vi "PicoScope3000aExampleStreamingAdvancedTrig.vi"() -> ()   [LabVIEW 2010]
doc: "This example demonstrates how to use the PicoScope Labview library to stream data from a PicoScope 5000 Series Device"
uses:
  <vilib>/Waveform/DWDTOps.llb/DWDT Analog to Digital.vi
  ps3000aWrap.dll
  PicoScope3000aLib/PicoScope3000aAnalogChannelSettings.ctl
  PicoScope3000aLib/PicoScope3000aDigitalChannelSettings.ctl
panel:
  in  "Write ChA to file":bool
  in  "Pulse Width Qualifier Conditions":T1 {"Condition Logic" items=["AND", "OR", "XOR"]}
  in  "Digital Port  0":T2 {"Direction Channel 7" items=["Don't Care", "Low", "High", "Rising", "Falling"]; "Direction Channel 6" items=["Don't Care", "Low", "High", "Rising", "Falling"]; "Direction Channel 5" items=["Don't Care", "Low", "High", "Rising", "Falling"]; "Direction Channel 4" items=["Don't Care", "Low", "High", "Rising", "Falling"]; "Direction Channel 3" items=["Don't Care", "Low", "High", "Rising", "Falling"]; "Direction Channel 2" items=["Don't Care", "Low", "High", "Rising", "Falling"]; "Direction Channel 1" items=["Don't Care", "Low", "High", "Rising", "Falling"]; "Direction Channel 0" items=["Don't Care", "Low", "High", "Rising", "Falling"]}
  in  "Pulse Width Qualifier Settings":T3={"Direction"=2, "Lower Limit"=0, "Upper Limit"=0, "Pulse Width Type"=0} {"Pulse Width Type" items=["None", "Less Than", "Greater Than", "In Range", "Out of Range"]; "Direction" items=["Rising"=2, "Falling"=3]}
  in  "Auto Trigger (ms)":i32=1000
  in  "Trigger Conditions":T4 {"Condition Logic" items=["AND", "OR", "XOR"]}
  in  "Channel B Trigger Properties":T5={"thresholdUpper"=0, "thresholdUpperHysteresis"=1024, "thresholdLower"=0, "thresholdLowerHysteresis"=1024, "Threshold Mode"=0, "Direction"=2, "Available"=FALSE} {"Direction" items=["Above / Inside", "Below / Outside", "Rising / Enter", "Falling / Exit", "Rising or Falling / Enter or Exit", "Above Lower", "Below Lower", "Rising Lower", "Falling Lower", "Positive Runt", "Negative Runt"]; "Threshold Mode" items=["Level", "Window"]}
  in  "Channel A Trigger Properties":T5={"thresholdUpper"=0, "thresholdUpperHysteresis"=1024, "thresholdLower"=0, "thresholdLowerHysteresis"=1024, "Threshold Mode"=0, "Direction"=2, "Available"=FALSE} {"Direction" items=["Above / Inside", "Below / Outside", "Rising / Enter", "Falling / Exit", "Rising or Falling / Enter or Exit", "Above Lower", "Below Lower", "Rising Lower", "Falling Lower", "Positive Runt", "Negative Runt"]; "Threshold Mode" items=["Level", "Window"]}
  in  "Port 0 Settings":T6={"Enabled"=FALSE, "Logic Level"=9830} {"Logic Level" items=["1.5V TTL"=9830, "2.5V CMOS"=16383]}
  in  "Channel A Settings":T7={"Enabled"=TRUE, "Coupling"=1, "Range"=6, "Analogue Offset"=0.0, "Bandwidth Limit"=0} {"Bandwidth Limit" items=["Full", "20MHz"]; "Range" items=["10 mV", "20 mV", "50 mV", "100 mV", "200 mV", "500 mV", "1 V", "2 V", "5 V", "10 V", "20 V", "50 V ", "100 V"]; "Coupling" items=["AC", "DC"]}
  out "Analog Channels":T8(graph)
  out "Raw Sample Interval (sec)":dbl=1.0000000130088963e-06 format="%#.5p"
  out "Max ADC value":i16
  out "Chunk time":u32
  out "Elapsed time":dbl
  in  "Data file":path=path "PicoScope3000aExampleStreaming ChA Data"
  out "size(s)":i32
  out "Queue depth":i32(graph)
  out "queue depth":i32
  in  "Buffer and Transfer Settings":T9={"startIndex"=0, "Samples"=1000000, "Down Sample Ratio"=1, "Down-Sample Mode"=0} {"Down-Sample Mode" items=["None"=0, "Aggregate"=1, "Decimate"=2, "Average"=4]; "Down Sample Ratio" step=1; "Samples" format="%_6p"}
  out "USB Powered":bool=TRUE
  out "USB 3.0 device on non-USB 3.0 Port":bool=TRUE
  out "TriggeredAt (In Buffer)":u32 format="%#.6p"
  out "TriggeredAt (Total samples)":u32 format="%#.6p"
  in  "Acquisition Settings":T10={"Auto Stop"=TRUE, "Desired Sample Interval"=1, "Pre-trigger Samples"=500000, "Post-trigger Samples"=500000, "Down-Sample Ratio"=1, "Down-Sample Mode"=0, "Time Units"=3} {"Time Units" items=["Nanoseconds (ns)"=2, "Microseconds (us)"=3, "Milliseconds (ms)"=4, "Seconds (s)"=5]; "Down-Sample Mode" items=["None"=0, "Aggregate"=1, "Decimate"=2, "Average"=4]; "Post-trigger Samples" format="%#.6p"; "Pre-trigger Samples" format="%#_6p"}
  out "Port 0":digitalwaveform(graph)={"t0"=timestamp(0 s since 1904-01-01), "dt"=1.0000000130088963e-06, "Y"={"transitions"=[], "data"=[]}}
  out "Triggered":bool
  out "DownSample Interval (sec)":dbl=1.0000000130088963e-06 format="%#.5p"
  out "Total Samples":u32 format="%#.6p"
  out "Auto Stopped":bool
  in  "Serial Number":string
  in  "Open Using Serial Number":bool
  out "Number of Samples per Capture":u32 format="%#.6p"
  in  "Apply  Settings":bool
  in  "stop":bool
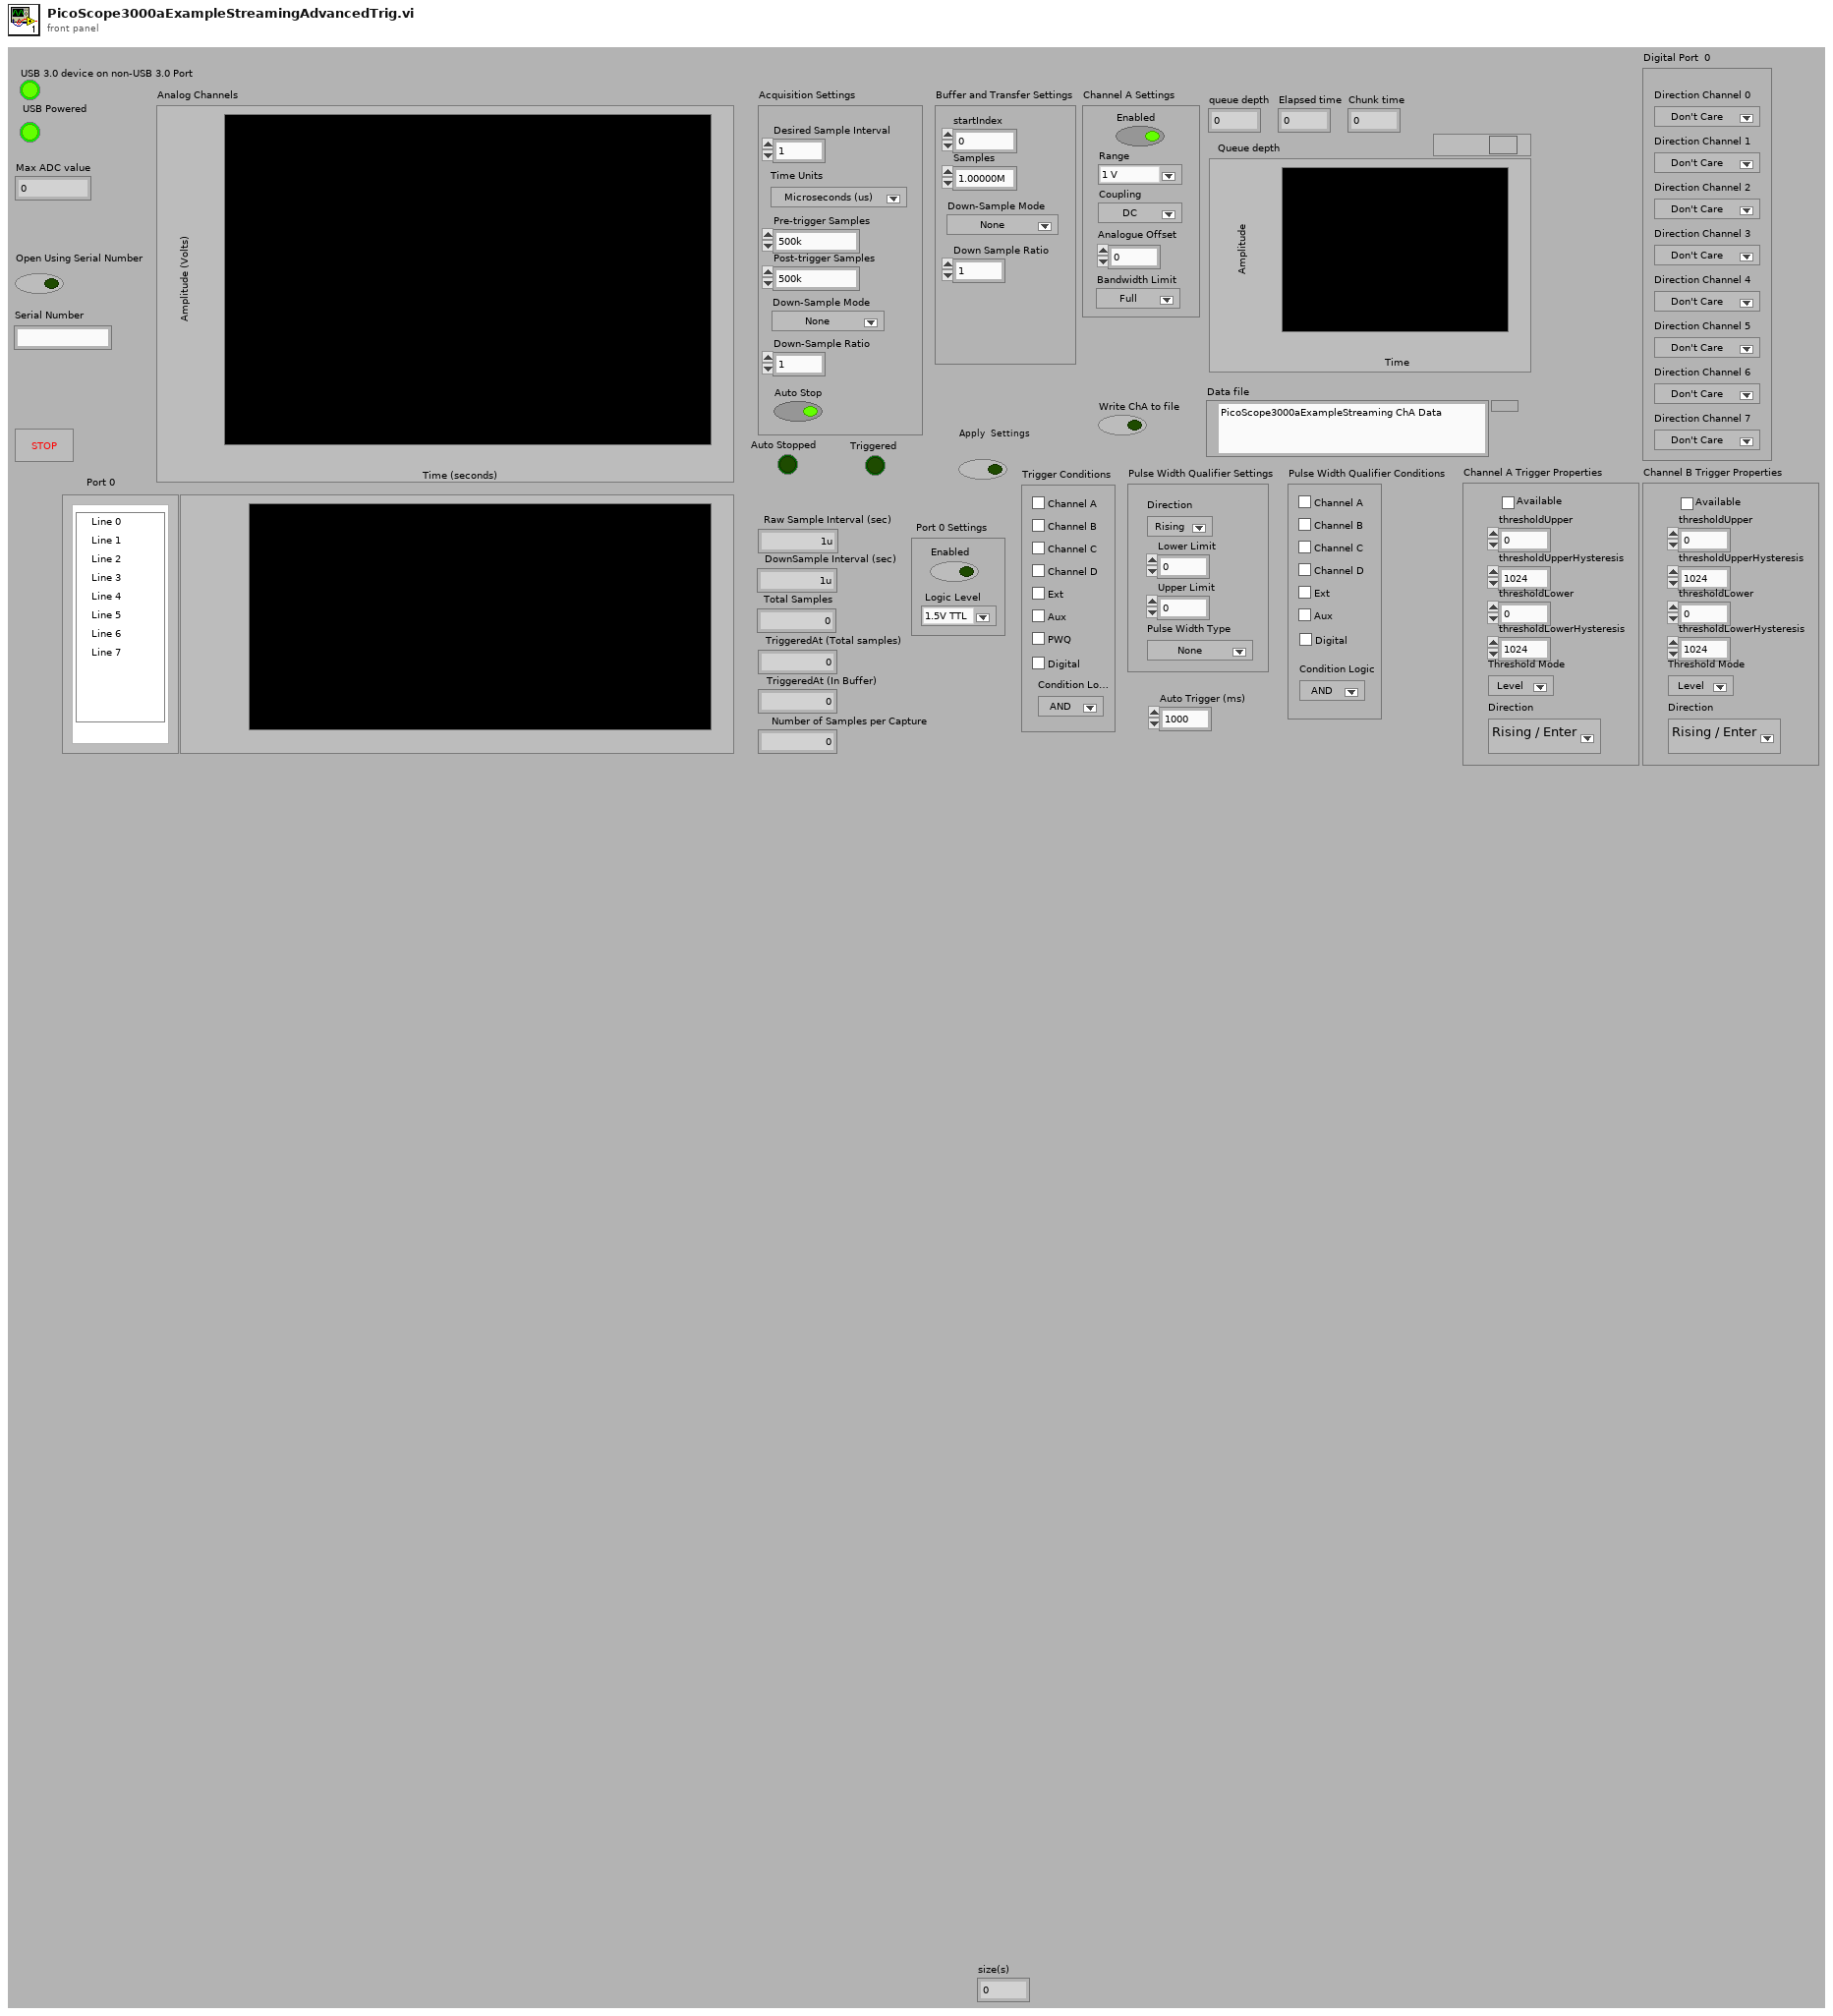
[diagram p1: front panel]
types:
  T1 = cluster{"Channel A":bool, "Channel B":bool, "Channel C":bool, "Channel D":bool, "Aux":bool, "Condition Logic":u16, "Ext":bool, "Digital":bool}
  T2 = cluster{"Direction Channel 0":u16, "Direction Channel 1":u16, "Direction Channel 2":u16, "Direction Channel 3":u16, "Direction Channel 4":u16, "Direction Channel 5":u16, "Direction Channel 6":u16, "Direction Channel 7":u16}
  T3 = cluster{"Direction":u32, "Lower Limit":u32, "Upper Limit":u32, "Pulse Width Type":u32}
  T4 = cluster{"Channel A":bool, "Channel B":bool, "Channel C":bool, "Channel D":bool, "Aux":bool, "PWQ":bool, "Condition Logic":u16, "Ext":bool, "Digital":bool}
  T5 = cluster{"thresholdUpper":i16, "thresholdUpperHysteresis":u16, "thresholdLower":i16, "thresholdLowerHysteresis":u16, "Threshold Mode":i32, "Direction":i32, "Available":bool}
  T6 = typedef "PicoScope3000aDigitalChannelSettings.ctl" = cluster{"Enabled":bool, "Logic Level":i16}
  T7 = typedef "PicoScope3000aAnalogChannelSettings.ctl" = cluster{"Enabled":bool, "Coupling":u32, "Range":u32, "Analogue Offset":sgl, "Bandwidth Limit":u32}
  T8 = cluster{i32, "DownSample Interval (sec)":dbl, "Data":dbl[]}
  T9 = cluster{"startIndex":u64, "Samples":u64, "Down Sample Ratio":u64, "Down-Sample Mode":u32}
  T10 = cluster{"Auto Stop":bool, "Desired Sample Interval":u32, "Pre-trigger Samples":u32, "Post-trigger Samples":u32, "Down-Sample Ratio":u32, "Down-Sample Mode":i32, "Time Units":u32}
  T11 = enum16{"open", "open or create", "create or replace", "create", "open (read-only)"}
  T12 = cluster{"Driver Version":string, "USB Version":string, "Hardware":string, "Variant":string, "Batch and Serial":string, "Cal Date":string, "Kernel Version":string, "Digital HW Version":string, "Analogue HW Version":string, "MSO":bool, "Number of channels":i16}
  T13 = cluster{"Channel A Buffer":i16[], "Channel B Buffer":i16[], "Channel C Buffer":i16[], "Channel D Buffer":i16[], "Channel E Buffer":i16[], "Channel F Buffer":i16[], "Channel G Buffer":i16[], "Channel H Buffer":i16[], "Port 0":i16[], "Port 1":i16[]}
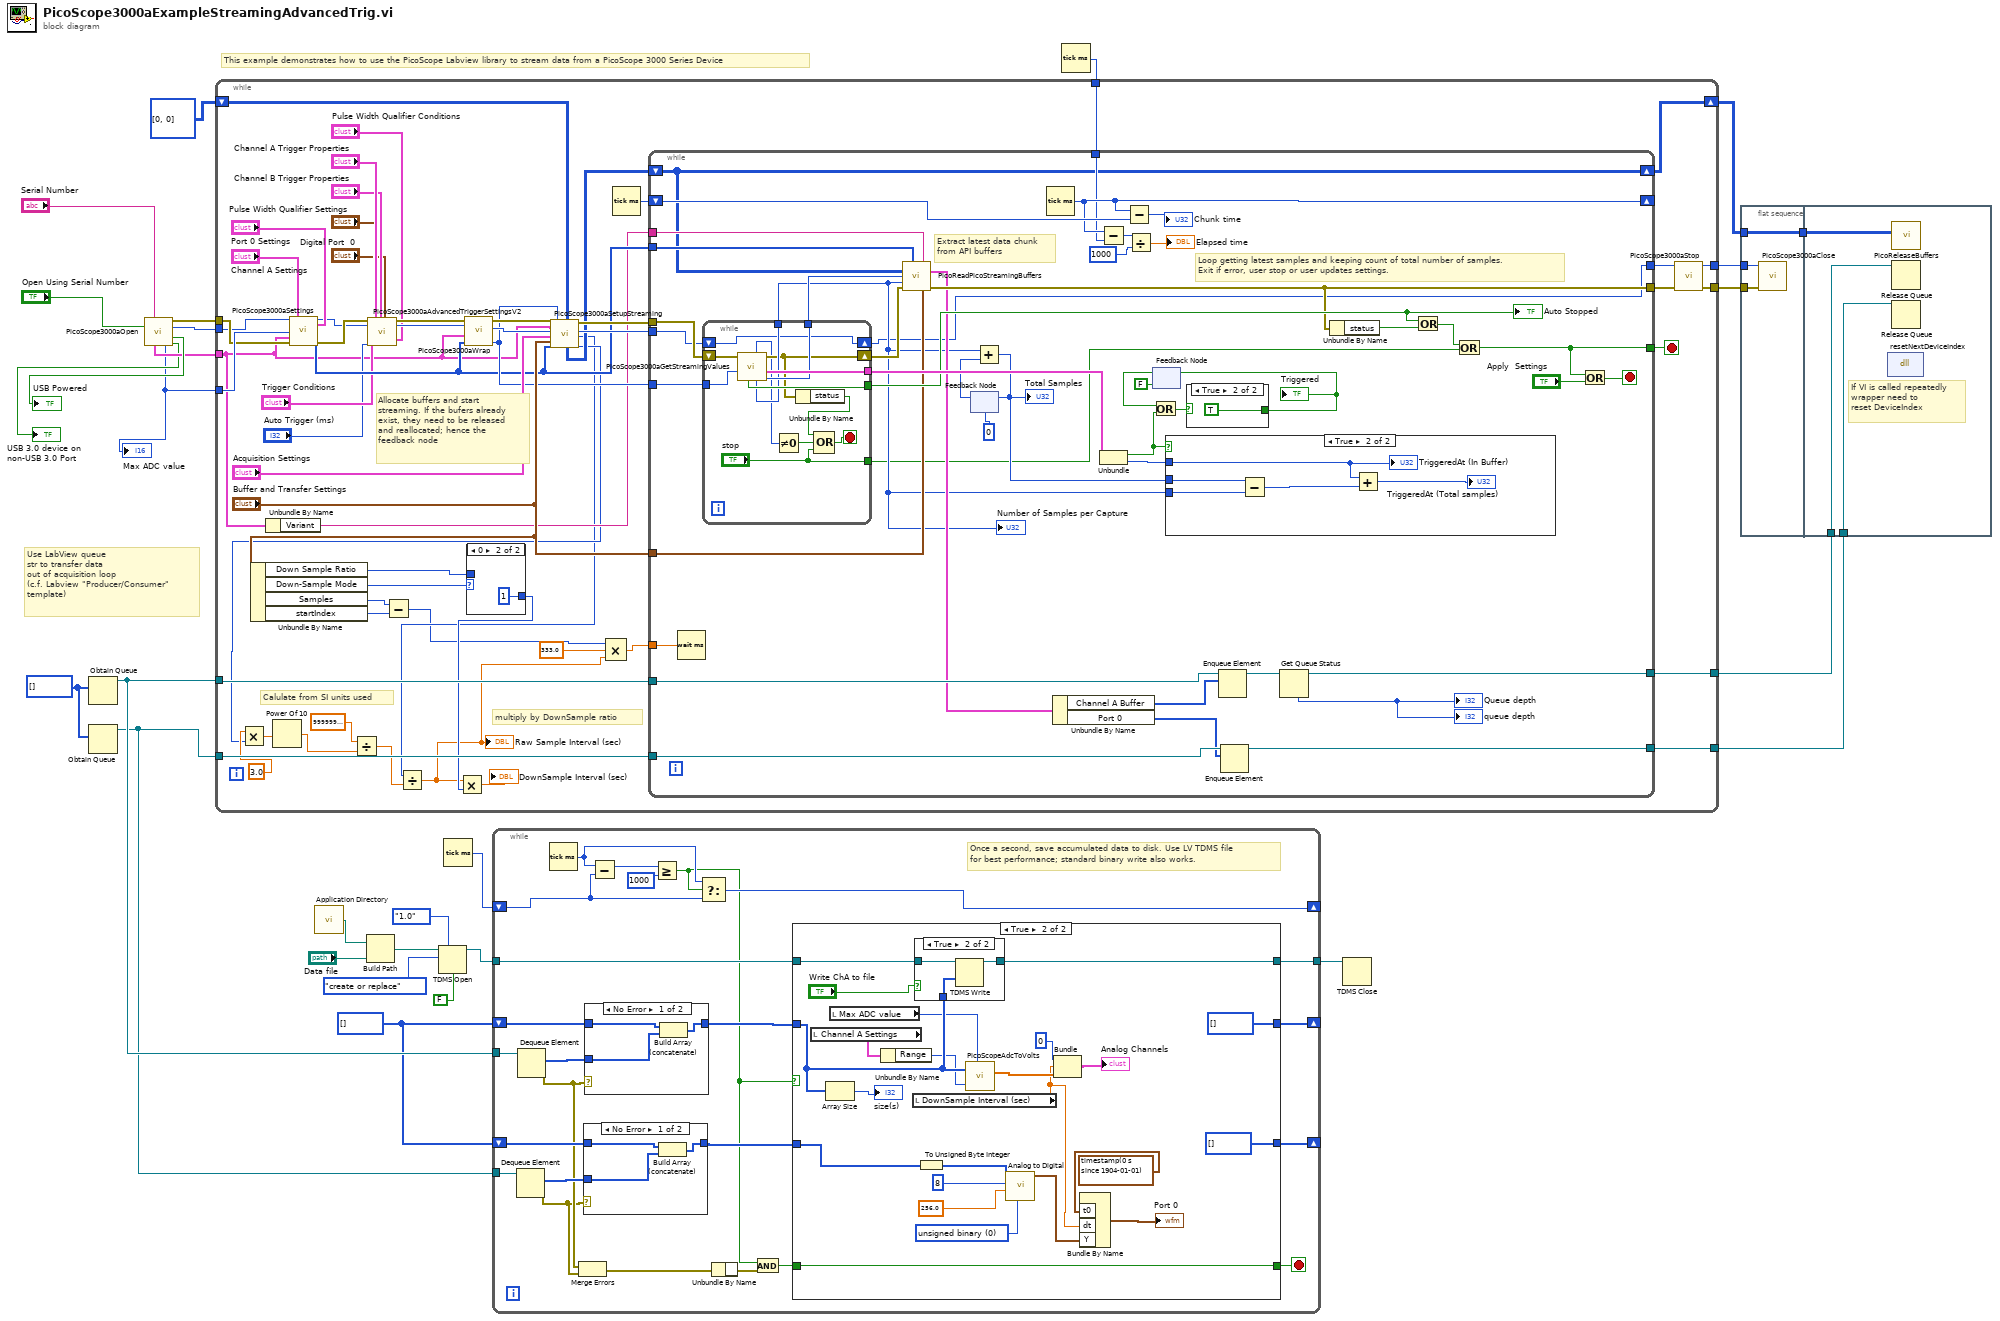
[diagram p0: block diagram]
diagram:
  w12 = i16[] [] ("History Data")
  w15 = i16[] [] ("History Data")
  # "Use LabView queue\nstr to transfer data\nout of acquisition loop\n(c.f. Labview \"Producer/Consumer\"\ntemplate)"
  # "This example demonstrates how to use the PicoScope Labview library to stream data from a PicoScope 3000 Series Device"
  n1 = Obtain Queue(element data type=w15) -> (queue out=w25:refnum<queue>)  [unwired: 4 in, 2 out]
  n2 = Obtain Queue(element data type=w15) -> (queue out=w13:refnum<queue>)  [unwired: 4 in, 2 out]
  n3 = call "PicoScope3000aOpen.vi"("Serial Number"="Serial Number", "Use Serial number"="Open Using Serial Number") -> ("error out"=w29:errorcluster, "handle"=w28:i16, "USB Powered"=→"USB Powered":bool, "Device Info"=w8:T12, "Max ADC value"=w6:i16, "USB 3.0 device on non-USB 3.0 Port"=→"USB 3.0 device on non-USB 3.0 Port":bool)  [unwired: 7 in, 1 out]
  "Max ADC value" <- w6
  n4 = call <vilib>:"Application Directory.vi"() -> ("Application Directory"=w9:path)
  n5 = Build Path(base path=w9, name or relative path="Data file") -> (appended path=w10:path)
  n6 = TDMS Open(6:FALSE ("disable buffering? (T)"), 7:enum16{"1.0", "2.0"}."1.0" ("file format version (2.0)"), 10:T11."create or replace" ("operation (0:open)"), 11:w10) -> (3:w19:refnum<k34>)  [unwired: 2 in, 1 out]
  n7 = Tick Count (ms)() -> (millisecond timer value=w21:u32)
  n8 = while {
    tunnel: w25 -> [w52]
    shift-right: [w44] -> _
    shift-left: w12 -> [w51]
    shift-right: [w46] -> _
    shift-left: w21 -> [w47]
    tunnel: w19 -> [w43]
    tunnel: [w42] -> w18
    tunnel: w13 -> [w40]
    shift-right: [w37] -> _
    shift-left: w12 -> [w39]
    stop <- w34 stop-if-true
    # "Once a second, save accumulated data to disk. Use LV TDMS file\nfor best performance; standard binary write also works."
    n9 = Dequeue Element(queue=w40) -> (element=w41:i16[], error out=w35:errorcluster)  [unwired: 2 in, 2 out]
    n10 = Dequeue Element(queue=w52) -> (element=w53:i16[], error out=w36:errorcluster)  [unwired: 2 in, 2 out]
    n11 = Tick Count (ms)() -> (millisecond timer value=w48:u32)
    n12 = Merge Errors(w36, w35) -> (w33:errorcluster)
    n13 = case shown="No Error" w35 {
      tunnel: w39 -> [w56 w57]
      tunnel: [w55 w57] -> w38
      tunnel: w41 -> [w54 _]
      frame No Error {
        n14 = Build Array (concatenate)(w56, w54) -> (w55:i16[])
      }
      frame Error {
      }
    }
    n15 = case shown="No Error" w36 {
      tunnel: w51 -> [w91 w92]
      tunnel: [w90 w92] -> w45
      tunnel: w53 -> [w89 _]
      frame No Error {
        n16 = Build Array (concatenate)(w91, w89) -> (w90:i16[])
      }
      frame Error {
      }
    }
    n17 = Subtract(x=w48, y=w47) -> (x-y=w50:u32)
    n18 = Greater Or Equal?(x=w50, y=u32 1000) -> (x >= y?=w31:bool)
    n19 = Select(t=w48, s=w31, f=w47) -> (s? t:f=w46:u32)
    n20 = And(x=w31) -> (y=w30:errorcluster, x .and. y?=w32:bool)
    n21 = Unbundle By Name(w33, w30) -> ()
    n22 = case shown="True" w31 {
      tunnel: w45 -> [w61 w80]
      tunnel: [w61 i16[] [] ("History Data")] -> w44
      tunnel: w43 -> [w60 w82]
      tunnel: [w60 w81] -> w42
      tunnel: w38 -> [w59 w67]
      tunnel: [w59 i16[] [] ("History Data")] -> w37
      tunnel: [w58 w63] -> w34
      tunnel: w32 -> [w58 w63]
      frame False {
      }
      frame True {
        w73 = u16 0 items=["unsigned binary", "offset binary", "2's complement"] ("data format (offset binary)")
        n23 = local read "Channel A Settings"() -> (w64:T7)
        n24 = Array Size(array=w80) -> (size(s)=→"size(s)":i32)
        n25 = local read "Max ADC value"() -> (w76:i16)
        n26 = Unbundle By Name(w64) -> ("Range"=w79:u32)
        n27 = local read "DownSample Interval (sec)"() -> (w68:dbl)
        n28 = case shown="True" "Write ChA to file" {
          tunnel: w82 -> [w85 w88]
          tunnel: [w85 w87] -> w81
          tunnel: w80 -> [_ w86]
          frame False {
          }
          frame True {
            n29 = TDMS Write(0:w88, 9:w86) -> (4:w87:refnum<k34>)  [unwired: 4 in, 3 out]
          }
        }
        n30 = To Unsigned Byte Integer(number=w67) -> (unsigned 8bit integer=w72:u8[])
        n31 = call "PicoScopeAdcToVolts.vi"("Max_adc"=w76, "Range Index"=w79, "Data"=w80) -> ("Data"=w77:dbl[])
        n32 = call-poly <vilib>:"Analog to Digital.vi"("data format (offset binary)"=w73, "full-scale range (pk-pk)"=256.0, "resolution (16 bit)"=8, "analog waveform"=w72) -> ("digital waveform"=w69:digitalwaveform)  [unwired: 4 in, 3 out]
        n33 = Bundle(0, "DownSample Interval (sec)"=w68, "Data"=w77) -> (→"Analog Channels":T8)  [unwired: 1 in]
        n34 = Bundle By Name("t0"=timestamp(0 s since 1904-01-01), "dt"=w68, "Y"=w69) -> (→"Port 0":digitalwaveform)  [unwired: 1 in]
      }
    }
  }
  n35 = Tick Count (ms)() -> (millisecond timer value=w24:u32)
  n36 = while {
    tunnel: w29 -> [w130]
    tunnel: w28 -> [w129]
    tunnel: w8 -> [w116]
    tunnel: w6 -> [w134]
    tunnel: [w141] -> w23
    tunnel: w25 -> [w140]
    tunnel: w24 -> [w138]
    tunnel: [w137] -> w14
    tunnel: w13 -> [w136]
    tunnel: [w112] -> w5
    tunnel: [w111] -> w4
    shift-right: [w108] -> w3
    shift-left: u64[][] [[0], [0]] ("Pointer array") -> [w110]
    stop <- w149 stop-if-true
    # "Calulate from SI units used"
    # "multiply by DownSample ratio"
    # "Allocate buffers and start\nstreaming. If the bufers already\nexist, they need to be released\nand reallocated; hence the\nfeedback node"
    n37 = Unbundle By Name("Buffer and Transfer Settings") -> ("Down Sample Ratio"=w144:u64, "Down-Sample Mode"=w145:u32, "Samples"=w107:u64, "startIndex"=w106:u64)
    n38 = Unbundle By Name(w116) -> ("Variant"=w115:string)
    n39 = call "PicoScope3000aSettings.vi"("handle in"=w129, "Channel A Settings"="Channel A Settings", "Port 0 Settings"="Port 0 Settings", "Max_adc"=w134, "Device Info"=w116, "error in"=w130) -> ("handle out"=w126:i16, "Enabled Array"=w128:i16[], "error out"=w127:errorcluster)  [unwired: 7 in]
    n40 = call "PicoScope3000aAdvancedTriggerSettingsV2.vi"("error in"=w127, "handle in"=w126, "Trigger Conditions"="Trigger Conditions", "Auto Trigger (ms)"="Auto Trigger (ms)", "Channel A Trigger Properties"="Channel A Trigger Properties", "Channel B Trigger Properties"="Channel B Trigger Properties", "Digital Port  0"="Digital Port  0", "Pulse Width Qualifier Conditions"="Pulse Width Qualifier Conditions", "Pulse Width Qualifier Settings"="Pulse Width Qualifier Settings") -> ("error out"=w125:errorcluster, "handle out"=w124:i16)  [unwired: 9 in]
    n41 = Subtract(x=w107, y=w106) -> (x-y=w95:u64)
    n42 = call "PicoScope3000aWrap.vi"("Enabled Array"=w128, "Device Info"=w116, "handle in"=w124, "error in (no error)"=w125) -> ("deviceIndex"=w131:u16, "handle out"=w132:i16, "error out"=w146:errorcluster)  [unwired: 1 in]
    n43 = case shown="0" w145 {
      tunnel: [w150 u32 1 ("Down-Sample Ratio")] -> w98
      tunnel: w144 -> [w150 _]
      frame Default {
      }
      frame 0 {
      }
    }
    n44 = call "PicoScope3000aSetupStreaming.vi"("error in"=w146, "Device Info"=w116, "handle in"=w132, "Acquisition Settings"="Acquisition Settings", "Buffer and Transfer Settings"="Buffer and Transfer Settings", "enabled array"=w128, "deviceIndex"=w131, "Pointers In"=w110) -> ("Pointer array"=w109:u64[][], "error out"=w147:errorcluster, "handle out"=w148:i16, "Sample Interval"=w97:u32, "sampleIntervalTimeUnits"=w99:u32)  [unwired: 7 in]
    n45 = Multiply(x=3.0, y=w99) -> (x*y=w104:dbl)
    n46 = Power Of 10(x=w104) -> (10^x=w103:dbl)
    n47 = Divide(x=sgl 1000000000000000.0 ("y"), y=w103) -> (x/y=w102:dbl)
    n48 = Divide(x=w97, y=w102) -> (x/y=w94:dbl)
    "Raw Sample Interval (sec)" <- w94
    n49 = Multiply(x=w94, y=w98) -> (x*y=→"DownSample Interval (sec)":dbl)
    n50 = Compound Arithmetic op=MULTIPLY(w95, 333.0 ("value"), w94) -> (w93:dbl)
    n51 = Tick Count (ms)() -> (millisecond timer value=w139:u32)
    n52 = while {
      tunnel: [w155] -> w113
      tunnel: [w196] -> w149
      tunnel: w148 -> [w156]
      tunnel: w147 -> [w181]
      tunnel: [w178] -> w114
      tunnel: "Buffer and Transfer Settings" -> [w180]
      tunnel: w128 -> [w177]
      tunnel: [w175] -> w141
      tunnel: w140 -> [w173]
      shift-right: [w167] -> _
      shift-left: w139 -> [w168]
      tunnel: w138 -> [w166]
      tunnel: w115 -> [w161]
      tunnel: [w152] -> w137
      tunnel: w136 -> [w160]
      tunnel: w131 -> [w157]
      shift-right: [w154] -> w108
      shift-left: w109 -> [w154]
      tunnel: w93 -> [w153]
      stop <- w195 stop-if-true
      # "Loop getting latest samples and keeping count of total number of samples. \nExit if error, user stop or user updates settings."
      # "Extract latest data chunk\nfrom API buffers"
      n53 = Wait (ms)(milliseconds to wait=w153) -> ()  [unwired: 1 out]
      n54 = while {
        tunnel: [w210] -> w194
        tunnel: [w209] -> w191
        tunnel: [w207] -> w163
        tunnel: [w206] -> w162
        shift-right: [w199] -> w155
        shift-left: w156 -> [w199]
        shift-right: [w205] -> w179
        shift-left: w181 -> [w208]
        tunnel: ["stop"] -> w158
        tunnel: w157 -> [w198]
        stop <- w201 stop-if-true
        n55 = call "PicoScope3000aGetStreamingValues.vi"("deviceIndex"=w198, "error in"=w208) -> ("Start Index"=w207:u32, "Trigger"=w210:cluster{bool, "triggeredAt (Total samples)":u32}, "error out"=w205:errorcluster, "Number of Samples"=w206:i32, "ready"=w204:i16, "Auto Stopped"=w209:bool)  [unwired: 4 in]
        n56 = Not Equal To 0?(x=w204) -> (x != 0?=w202:bool)
        n57 = Unbundle By Name(w205) -> ("status"=w203:bool)
        n58 = Compound Arithmetic op=OR(w203, w202, "stop") -> (w201:bool)
      }
      "Number of Samples per Capture" <- w162
      "Auto Stopped" <- w191
      n59 = call "PicoReadPicoStreamingBuffers.vi"("enabled array"=w177, "Buffer and Transfer Settings"=w180, "Variant"=w161, "Pointer array"=w154, "Offset Index"=w163, "Number of Samples"=w162, "error in (no error)"=w179) -> ("Buffers (Max or non-aggregated)"=w172:T13, "error out"=w178:errorcluster)  [unwired: 6 in, 1 out]
      n60 = feedback #1(u32 0) -> (w187:u32)
      n61 = Add(x=w162, y=w187) -> (x+y=w185:u32)
      "Total Samples" <- w185
      n62 = feedback-in #1(w185) -> ()
      n63 = Tick Count (ms)() -> (millisecond timer value=w167:u32)
      n64 = Unbundle By Name(w172) -> ("Channel A Buffer"=w164:i16[], "Port 0"=w159:i16[])
      n65 = Subtract(x=w167, y=w166) -> (x-y=w171:u32)
      n66 = Unbundle(w194) -> (w183:bool, "triggeredAt (Total samples)"=w182:u32)
      n67 = Subtract(x=w167, y=w168) -> (x-y=→"Chunk time":u32)
      n68 = Divide(x=w171, y=u32 1000) -> (x/y=→"Elapsed time":dbl)
      n69 = feedback #2(FALSE) -> (w189:bool)
      n70 = Or(x=w189, y=w183) -> (x .or. y?=w186:bool)
      n71 = case shown="True" w183 {
        tunnel: w162 -> [_ w211]
        tunnel: w185 -> [_ w215]
        tunnel: w182 -> [_ w213]
        frame False {
        }
        frame True {
          n72 = Subtract(x=w215, y=w211) -> (x-y=w214:u32)
          n73 = Add(x=w213, y=w214) -> (x+y=→"TriggeredAt (Total samples)":u32)
          "TriggeredAt (In Buffer)" <- w213
        }
      }
      n74 = case shown="True" w186 {
        selector: w186 -> [w216 _]
        tunnel: [w216 TRUE] -> w184
        frame False {
        }
        frame True {
        }
      }
      "Triggered" <- w184
      n75 = feedback-in #2(w184) -> ()
      n76 = Enqueue Element(queue=w173, element=w164) -> (queue out=w174:refnum<queue>)  [unwired: 2 in, 2 out]
      n77 = Enqueue Element(queue=w160, element=w159) -> (queue out=w152:refnum<queue>)  [unwired: 2 in, 2 out]
      n78 = Get Queue Status(queue=w174) -> (queue out=w175:refnum<queue>, # elements in queue=→"queue depth" →"Queue depth":i32)  [unwired: 2 in, 6 out]
      n79 = Unbundle By Name(w178) -> ("status"=w193:bool)
      n80 = Or(x=w191, y=w193) -> (x .or. y?=w192:bool)
      n81 = Or(x=w192, y=w158) -> (x .or. y?=w196:bool)
      n82 = Or(x=w196, y="Apply  Settings") -> (x .or. y?=w195:bool)
    }
    n83 = call "PicoScope3000aStop.vi"("error in (no error)"=w114, "handle in"=w113) -> ("error out"=w112:errorcluster, "handle out"=w111:i16)  [unwired: 8 in]
  }
  n84 = TDMS Close(11:w18) -> ()  [unwired: 1 in, 2 out]
  n85 = flat-sequence {
    tunnel: w5 -> [w220]
    tunnel: w4 -> [w219]
    tunnel: w3 -> [w218]
    tunnel: [w218] -> w1
    tunnel: w23 -> [w223]
    tunnel: w14 -> [w222]
    tunnel: w1 -> [w221]
    frame #0 {
      n86 = call "PicoScope3000aClose.vi"("error in (no error)"=w220, "handle in"=w219) -> ()  [unwired: 8 in, 2 out]
    }
    frame #1 {
      # "If VI is called repeatedly\nwrapper need to\nreset DeviceIndex"
      n87 = dll-call lib="ps3000aWrap.dll" fn="resetNextDeviceIndex"() -> ()  [unwired: 4 in, 2 out]
      n88 = call "PicoReleaseBuffers.vi"("Pointer array"=w221) -> ()  [unwired: 9 in, 2 out]
      n89 = Release Queue(queue=w223) -> ()  [unwired: 2 in, 3 out]
      n90 = Release Queue(queue=w222) -> ()  [unwired: 2 in, 3 out]
    }
  }
